vi "Compila da file.vi"(10 "appended array":refnum<vi>[](array[refnum]), 11 "start path":path=path "") -> (3 "Array":string[](array[string]))   [LabVIEW 2019]
uses:
  read_excel_values.llb/GetXL_CellValues_2D_String.vi
panel:
  out "data":string[][](array[string])
  in  "Start":cluster{"Column":i32, "Row":i32}={"Column"=1, "Row"=1}
  in  "End":cluster{"Column":i32, "Row":i32}={"Column"=30, "Row"=2}
  out "error out 2":errorcluster
  in  "Sheet":i32=1
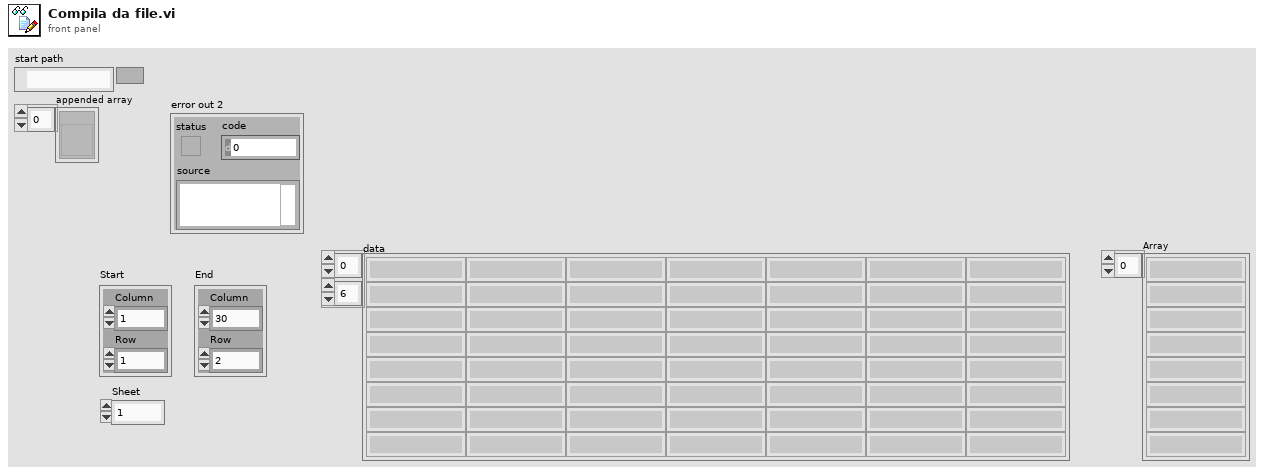
[diagram p1: front panel]
types:
  T1 = cluster{"Excel._Application":refnum<k7>, "Workbooks":refnum<k7>}
  T2 = cluster{"Excel._Application":refnum<k7>, "Workbooks":refnum<k7>, "Open":refnum<k7>}
  T3 = cluster{"Excel._Application":refnum<k7>, "Workbooks":refnum<k7>, "Open":refnum<k7>, "Worksheets":refnum<k7>, "Excel._Worksheet":refnum<k7>}
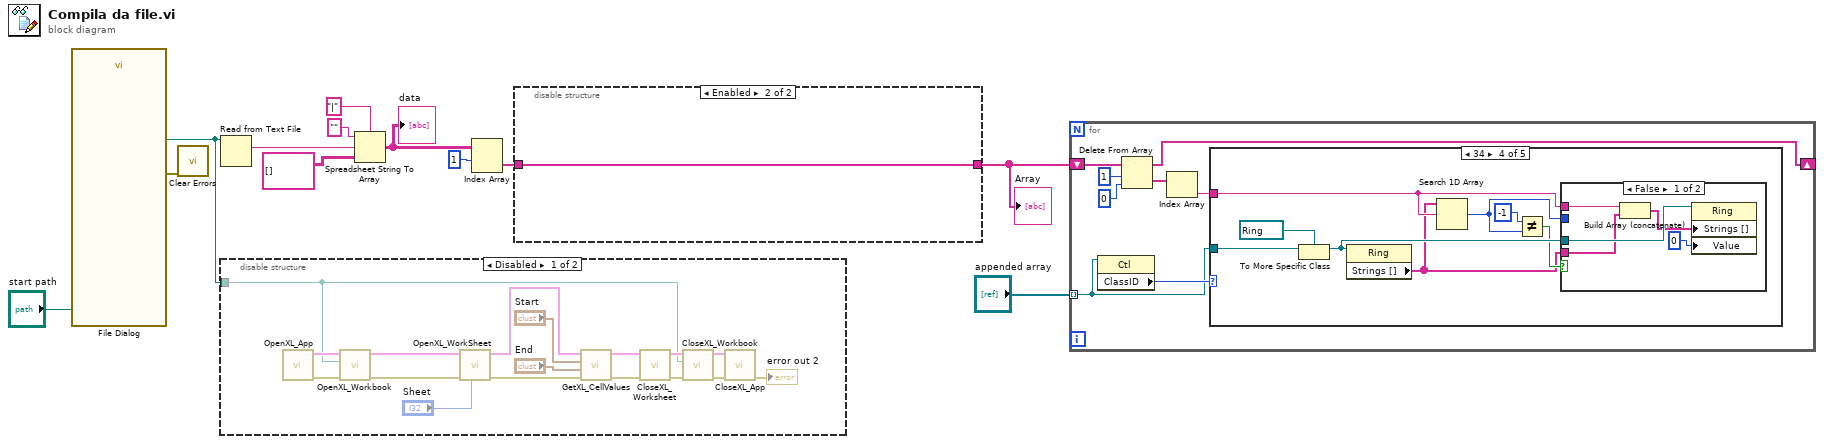
[diagram p0: block diagram]
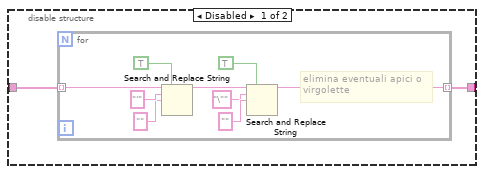
[diagram p2: hidden frame]
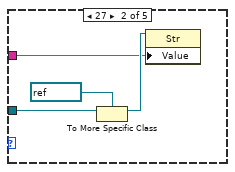
[diagram p5: hidden frame]
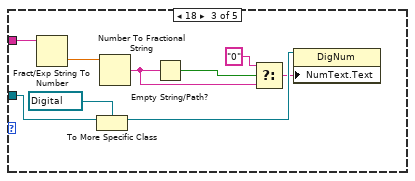
[diagram p6: hidden frame]
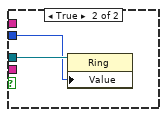
[diagram p7: hidden frame]
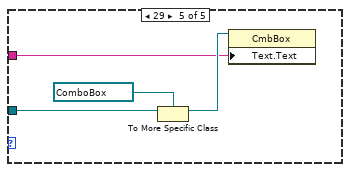
[diagram p8: hidden frame]
diagram:
  n1 = call "File Dialog"("start path"="start path") -> ("selected path"=w2:path, "error out"=w12:errorcluster)  [unwired: 6 in, 7 out]
  n2 = call <vilib>:"Clear Errors.vi"("error in (no error)"=w12) -> ()  [unwired: 5 in, 2 out]
  n3 = Read from Text File(file (use dialog)=w2) -> (text=w6:string)  [unwired: 3 in, 3 out]
  n4 = disable-structure shown="Disabled" {
    disable-tunnel: w2 -> [w13 _]
    frame Disabled {
      n5 = call "OpenXL_App.vi"() -> ("error out"=w22:errorcluster, "Refnum Cluster"=w21:T1)  [unwired: 10 in]
      n6 = call "OpenXL_Workbook.vi"("error in"=w22, "path"=w13, "Refnum Cluster In"=w21) -> ("error out"=w24:errorcluster, "Refnum Cluster Out"=w23:T2)  [unwired: 7 in]
      n7 = call "OpenXL_WorkSheet.vi"("Sheet"="Sheet", "error in (no error)"=w24, "Refnum Cluster In"=w23) -> ("error out"=w15:errorcluster, "Refnum Cluster Out"=w14:T3)  [unwired: 7 in]
      n8 = call-poly "GetXL_CellValues.vi"("error in"=w15, "End"="End", "Start"="Start", "Refnum Cluster In"=w14) -> ("error out"=w26:errorcluster, "Refnum Cluster Out"=w25:T3)  [unwired: 5 in, 1 out]
      n9 = call "CloseXL_Worksheet.vi"("error in (no error)"=w26, "Refnum Cluster In"=w25) -> ("error out"=w28:errorcluster, "Refnum Cluster Out"=w27:T2)  [unwired: 8 in]
      n10 = call "CloseXL_Workbook.vi"("error in (no error)"=w28, "path"=w13, "Refnum Cluster In"=w27) -> ("error out"=w17:errorcluster, "Refnum Cluster Out"=w16:T1)  [unwired: 7 in]
      n11 = call "CloseXL_App.vi"("error in (no error)"=w17, "Refnum Cluster In"=w16) -> ("error out"=→"error out 2":errorcluster)  [unwired: 9 in]
    }
    frame Enabled {
    }
  }
  n12 = Spreadsheet String To Array(delimiter (Tab)="|", format string="", spreadsheet string=w6, array type (2D Dbl)=string[][] []) -> (array=w1:string[][])
  "data" <- w1
  n13 = Index Array(array=w1, index (row)=1) -> (element=w9:string[])  [unwired: 1 in]
  n14 = disable-structure shown="Enabled" {
    disable-tunnel: w9 -> [w31 w41]
    disable-tunnel: [w30 w41] -> w8
    frame Disabled {
      n15 = for {
        tunnel: w31 -> [w40] mode=indexing
        tunnel: [w32] -> w30 mode=indexing
        # "elimina eventuali apici o\nvirgolette"
        n16 = Search and Replace String(replace all?=TRUE ("replace all? (F)"), input string=w40, search string="'", replace string="" ("replace string (\"\")")) -> (result string=w33:string)  [unwired: 4 in, 3 out]
        n17 = Search and Replace String(replace all?=TRUE ("replace all? (F)"), input string=w33, search string="\"", replace string="" ("replace string (\"\")")) -> (result string=w32:string)  [unwired: 4 in, 3 out]
      }
    }
    frame Enabled {
    }
  }
  "Array" <- w8
  n18 = for {
    tunnel: "appended array" -> [w48] mode=indexing
    shift-right: [w46] -> _
    shift-left: w8 -> [w47]
    n19 = property class="Ctl"(reference=w48) -> ("ClassID"=w49:u32)  [unwired: 1 in, 2 out]
    n20 = Delete From Array(array=w47, length=1, index=0) -> (deleted portion=w45:string[], array with subset deleted=w46:string[])
    n21 = Index Array(array=w45) -> (element=w43:string)  [unwired: 1 in]
    n22 = case shown="34" w49 {
      tunnel: w48 -> [_ w52 w62 w69 w81]
      tunnel: w43 -> [_ w50 w55 w64 w78]
      frame 0, Default {
      }
      frame 27 {
        n23 = To More Specific Class(target class=refnum<vi> refnum ("String"), reference=w52) -> (specific class reference=w51:refnum<vi>)  [unwired: 1 in, 1 out]
        n24 = property class="Str"(reference=w51, "Value"=w50) -> ()  [unwired: 1 in, 2 out]
      }
      frame 18 {
        n25 = Fract/Exp String To Number(string=w55) -> (number=w56:dbl)  [unwired: 3 in, 1 out]
        n26 = To More Specific Class(target class=refnum<vi> refnum ("Numeric Control"), reference=w62) -> (specific class reference=w60:refnum<vi>)  [unwired: 1 in, 1 out]
        n27 = Number To Fractional String(number=w56) -> (F-format string=w54:string)  [unwired: 3 in]
        n28 = Empty String/Path?(string/path=w54) -> (empty?=w59:bool)
        n29 = Select(t="0", s=w59, f=w54) -> (s? t:f=w57:string)
        n30 = property class="DigNum"(reference=w60, "NumText.Text"=w57) -> ()  [unwired: 1 in, 2 out]
      }
      frame 34 {
        n31 = To More Specific Class(target class=refnum<vi> refnum ("Menu Ring"), reference=w69) -> (specific class reference=w68:refnum<vi>)  [unwired: 1 in, 1 out]
        n32 = property class="Ring"(reference=w68) -> ("Strings []"=w63:string[])  [unwired: 1 in, 2 out]
        n33 = Search 1D Array(1D array=w63, element=w64) -> (index of element=w66:i32)  [unwired: 1 in]
        n34 = Not Equal?(x=-1, y=w66) -> (x != y?=w67:bool)
        n35 = case shown="False" w67 {
          tunnel: w68 -> [w75 w77]
          tunnel: w66 -> [_ w76]
          tunnel: w64 -> [w73 _]
          tunnel: w63 -> [w74 _]
          frame False {
            n36 = Build Array (concatenate)(w73, w74) -> (w72:string[])
            n37 = property class="Ring"(reference=w75, "Strings []"=w72, "Value"=0) -> ()  [unwired: 1 in, 2 out]
          }
          frame True {
            n38 = property class="Ring"(reference=w77, "Value"=w76) -> ()  [unwired: 1 in, 2 out]
          }
        }
      }
      frame 29 {
        n39 = To More Specific Class(target class=refnum<vi> refnum ("FILE TARATURA"), reference=w81) -> (specific class reference=w80:refnum<vi>)  [unwired: 1 in, 1 out]
        n40 = property class="CmbBox"(reference=w80, "Text.Text"=w78) -> ()  [unwired: 1 in, 2 out]
      }
    }
  }
